vi "4Pi 4Pi Modes - Coefficients  AE.vi"(0 "Coefficients In":cluster{"Mode":string, "Amplitude":dbl}[](array[cluster]), 2 "Action":T1) -> (4 "Coefficients Out":cluster{"Mode":string, "Amplitude":dbl}[](array[cluster]))   [LabVIEW 2016]
uses:
  4Pi 4Pi Modes - Controls/4Pi 4Pi Modes - Standard Action.ctl
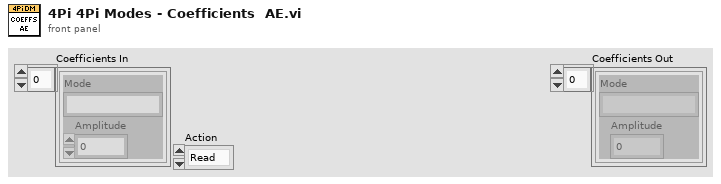
[diagram p1: front panel]
types:
  T1 = typedef "4Pi 4Pi Modes - Standard Action.ctl" = enum16{"Read", "Write"}
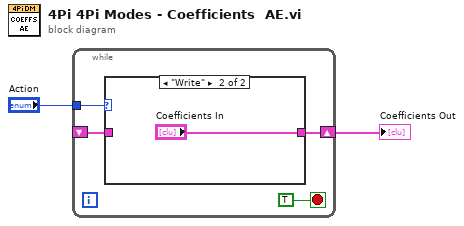
[diagram p0: block diagram]
diagram:
  n1 = while {
    tunnel: "Action" -> [w6]
    shift-right: [w5] -> w1
    shift-left: _ -> [w3]
    stop <- TRUE stop-if-true
    n2 = case shown="\"Write\"" w6 {
      tunnel: [w7 "Coefficients In"] -> w5
      tunnel: w3 -> [w7 _]
      frame "Read", Default {
      }
      frame "Write" {
      }
    }
  }
  "Coefficients Out" <- w1
